vi "Read Data Bits.vi"(8 "error in (no error)":errorcluster, 11 "ASCII data unit in":refnum<class "ASCII Data Unit.lvclass">) -> (0 "error out":errorcluster, 2 "data bits":u16=7, 3 "ASCII data unit out":refnum<class "ASCII Data Unit.lvclass">)   [LabVIEW 2020, in "SubVIs.lvlib" / "ASCII Data Unit.lvclass"]
doc: "Acts as a constant, and provides a way for the serial slave to properly configure the serial interface. 7 bits in this case."
uses:
  <vilib>/Modbus/subvis/Transmission Data Unit (ADU)/ASCII Data Unit/ASCII Data Unit.lvclass
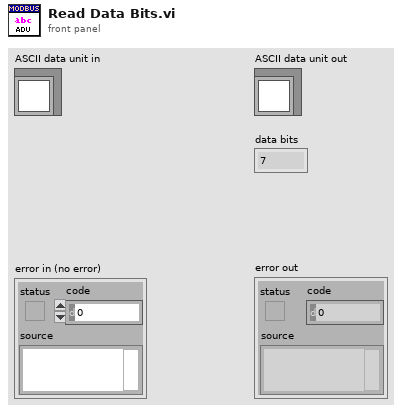
[diagram p1: front panel]
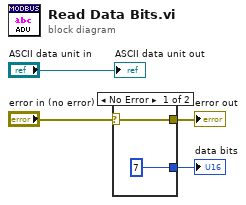
[diagram p0: block diagram]
diagram:
  n1 = case shown="No Error" "error in (no error)" {
    selector: "error in (no error)" -> [w5 w7]
    tunnel: [u16 7 ("data bits") _] -> w3
    tunnel: [w5 w7] -> w1
    frame No Error {
    }
    frame Error {
    }
  }
  "error out" <- w1
  "data bits" <- w3
  "ASCII data unit out" <- "ASCII data unit in"
